vi "Apply Config.vi"(8 "error in (no error)":errorcluster, 11 "AW Config in":refnum<class "AW Config.lvclass">) -> (0 "error out":errorcluster, 3 "AW Config out":refnum<class "AW Config.lvclass">)   [LabVIEW 2023, in "PXI-5441.lvlib" / "AW Config.lvclass"]
uses:
  AW Config.lvclass
  AW Config.lvclass/AW Config.ctl
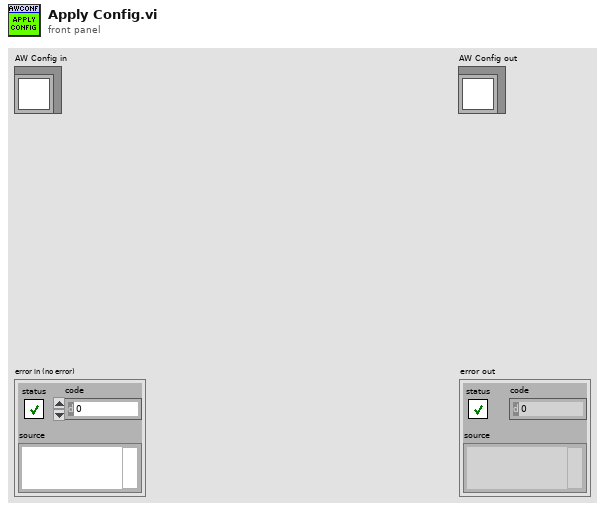
[diagram p1: front panel]
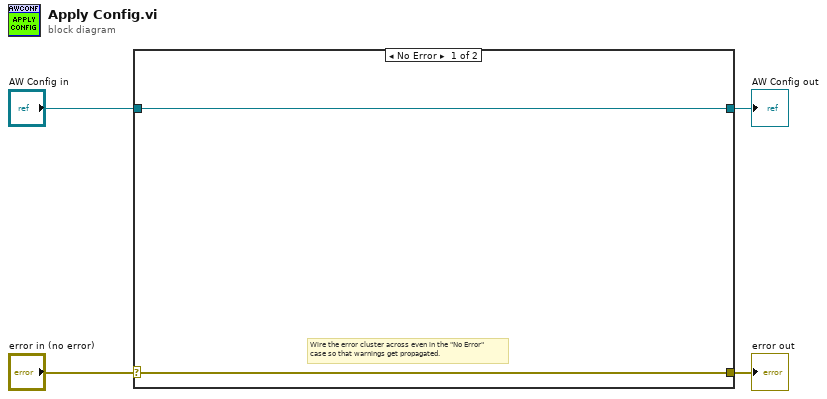
[diagram p0: block diagram]
diagram:
  n1 = case shown="No Error" "error in (no error)" {
    selector: "error in (no error)" -> [w5 w8]
    tunnel: [w5 w8] -> w3
    tunnel: [w6 w7] -> w1
    tunnel: "AW Config in" -> [w6 w7]
    frame No Error {
      # "Wire the error cluster across even in the \"No Error\"\ncase so that warnings get propagated."
    }
    frame Error {
    }
  }
  "error out" <- w3
  "AW Config out" <- w1
